vi "UIdisplay.vi"(8 "error in (no error)":errorcluster, 9 "Step":i32, 10 "result":bool, 11 "Vaule":string) -> (0 "error out":errorcluster)   [LabVIEW 2017]
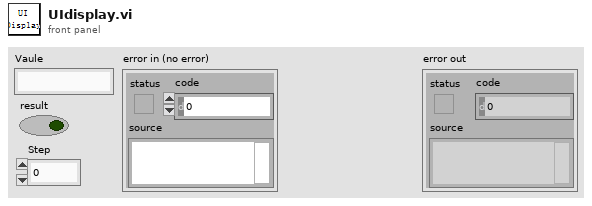
[diagram p1: front panel]
types:
  T1 = cluster{"Vaule":string, "result":bool, "Step":i32}
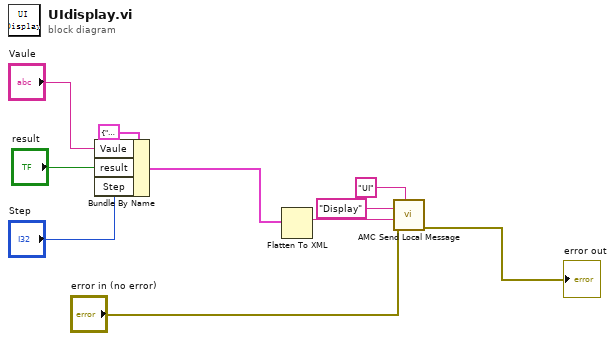
[diagram p0: block diagram]
diagram:
  n1 = Bundle By Name(cluster=T1 {"Vaule"="", "result"=FALSE, "Step"=0} ("Vaule"), "Vaule"="Vaule", "result"="result", "Step"="Step") -> (w4:T1)
  n2 = Flatten To XML(anything=w4) -> (xml string=w8:string)
  n3 = call "AMC Send Local Message.vi"("Process (\"\" - local)"="UI" ("Process (\"\" - local)"), "error in (no error)"="error in (no error)", "Message Value"=w8, "Message Name"="Display") -> ("error out"=→"error out":errorcluster)  [unwired: 6 in, 1 out]
